vi "FPGA - Split Audio.vi"(1 "Enable":T1={"Track 0"=TRUE, "Track 1"=TRUE, "Track 2"=TRUE, "Track 3"=TRUE}, 2 "U64 Audio In":u64) -> (5 "Track 0 Out":u16, 6 "Track 1 Out":u16, 7 "Track 2 Out":u16, 8 "Track 3 Out":u16)   [LabVIEW 2014]
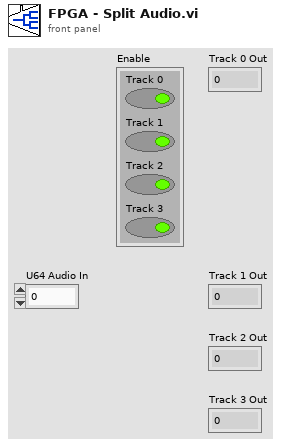
[diagram p1: front panel]
types:
  T1 = cluster{"Track 0":bool, "Track 1":bool, "Track 2":bool, "Track 3":bool}
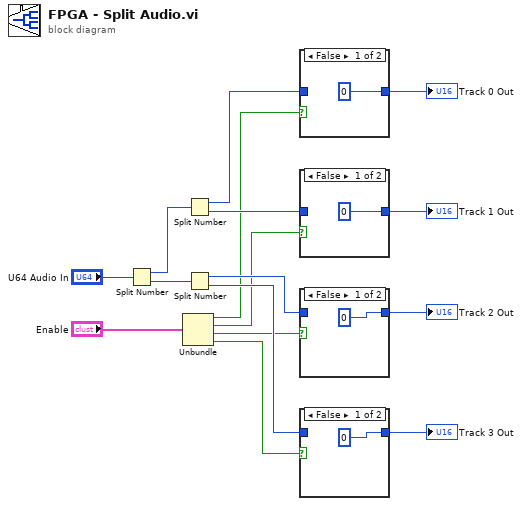
[diagram p0: block diagram]
diagram:
  n1 = Split Number(x="U64 Audio In") -> (hi(x)=w15:u32, lo(x)=w14:u32)
  n2 = Unbundle("Enable") -> ("Track 0"=w4:bool, "Track 1"=w3:bool, "Track 2"=w2:bool, "Track 3"=w1:bool)
  n3 = Split Number(x=w15) -> (hi(x)=w12:u16, lo(x)=w10:u16)
  n4 = Split Number(x=w14) -> (hi(x)=w9:u16, lo(x)=w8:u16)
  n5 = case shown="False" w4 {
    tunnel: w12 -> [_ w18]
    tunnel: [u16 0 w18] -> w11
    frame False {
    }
    frame True {
    }
  }
  "Track 0 Out" <- w11
  n6 = case shown="False" w3 {
    tunnel: w10 -> [_ w20]
    tunnel: [u16 0 w20] -> w7
    frame False {
    }
    frame True {
    }
  }
  "Track 1 Out" <- w7
  n7 = case shown="False" w2 {
    tunnel: w9 -> [_ w22]
    tunnel: [u16 0 w22] -> w6
    frame False {
    }
    frame True {
    }
  }
  "Track 2 Out" <- w6
  n8 = case shown="False" w1 {
    tunnel: w8 -> [_ w24]
    tunnel: [u16 0 w24] -> w5
    frame False {
    }
    frame True {
    }
  }
  "Track 3 Out" <- w5
